vi "Process XML Node.vi"(8 "error in (no error)":errorcluster, 11 "node in":refnum<k20>) -> (0 "error out":errorcluster, 2 "Attribute":refnum<class "Attribute.lvclass">, 3 "node out":refnum<k20>)   [LabVIEW 2023, in "VILab.lvlib"]
uses:
  VILab.lvlib
  Classes/Attribute/Attribute.lvclass
  Classes/Data Item/Data Item.lvclass/Data Item.ctl
  Classes/Element/Element.lvclass/Element.ctl
  Classes/Attribute/Attribute.lvclass/Attribute.ctl
  Classes/Element Array/Element Array.lvclass
  Classes/Element/Element.lvclass
  Classes/Reference/Reference.lvclass
  Classes/Reference/Create Reference.vi
  Classes/Data Item/Data Item.lvclass
  Classes/Attribute/Create Attribute (Data Item).vi
  <vilib>/xml/NI_XML.lvlib
  <resource>/objmgr/DOMUserDefRef.rc
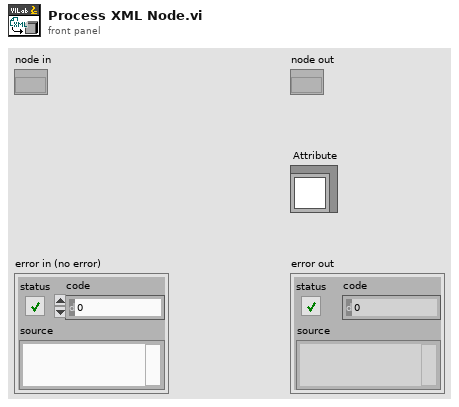
[diagram p1: front panel]
types:
  T1 = cluster{"class":string, "uid":string, "Attributes":refnum<class "Attribute.lvclass">[], "Array?":bool}
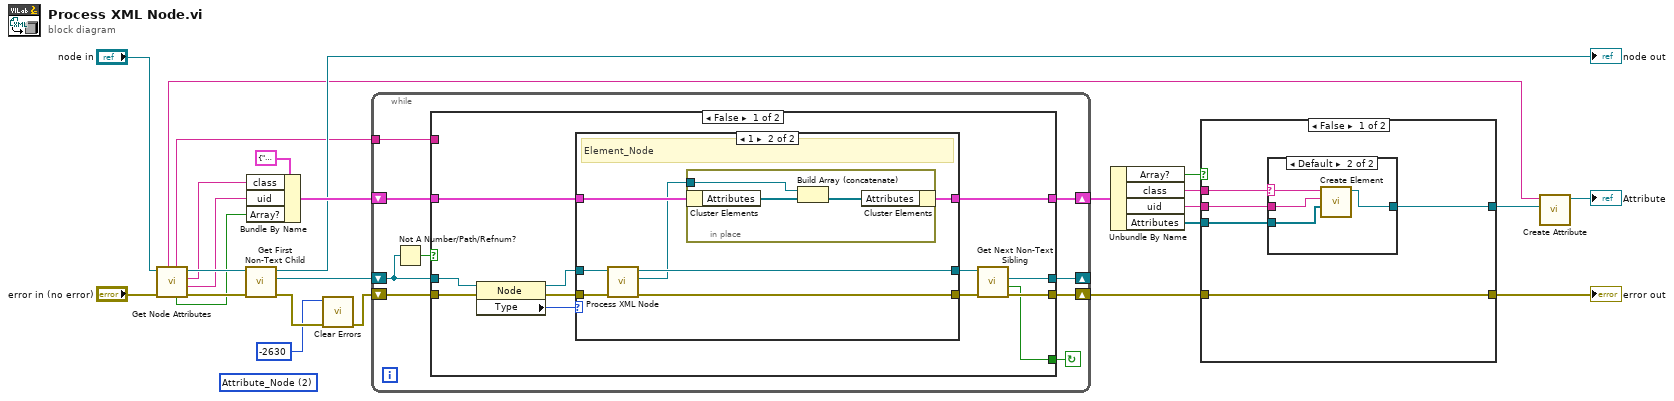
[diagram p0: block diagram]
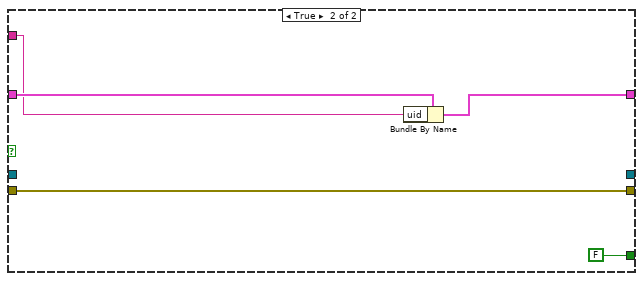
[diagram p3: hidden frame]
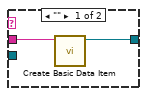
[diagram p4: hidden frame]
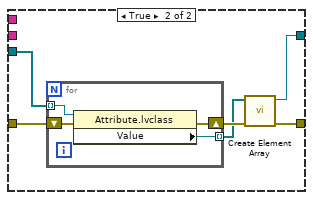
[diagram p5: hidden frame]
diagram:
  (unwired) 2 items=["Element_Node"=1, "Attribute_Node"=2, "Text_Node"=3, "CDATASection_Node"=4, "EntityReference_Node"=5, "Entity_Node"=6, "ProcessingInstruction_Node"=7, "Comment_Node"=8, "Document_Node"=9, "DocumentType_Node"=10, "DocumentFragment_Node"=11, "Notation_Node"=12] ("Node Type")
  n1 = call "Get Node Attributes.vi"("error in (no error)"="error in (no error)", "node in"="node in") -> ("error out"=w25:errorcluster, "uid"=w12:string, "class"=w13:string, "node out"=w15:refnum<k20>, "Array?"=w8:bool, "Value"=w1:string, "Name"=w2:string)  [unwired: 3 in]
  n2 = call <vilib>:"Get First Non-Text Child.vi"("error in (no error)"=w25, "node in"=w15) -> ("error out"=w23:errorcluster, "child node"=w19:refnum<k20>, "node out"=→"node out":refnum<k20>)  [unwired: 6 in, 1 out]
  n3 = Bundle By Name(cluster=T1 {"class"="", "uid"="", "Attributes"=[], "Array?"=FALSE}, "class"=w13, "uid"=w12, "Array?"=w8) -> (w11:T1)
  n4 = call <vilib>:"Clear Errors.vi"("error in (no error)"=w23, "specific error code to clear (0: all)"=-2630) -> ("error out"=w22:errorcluster)  [unwired: 4 in, 1 out]
  n5 = while {
    shift-right: [w30] -> w18
    shift-left: w11 -> [w31]
    shift-right: [w34] -> w21
    shift-left: w22 -> [w33]
    shift-right: [w29] -> _
    shift-left: w19 -> [w27]
    tunnel: w1 -> [w26]
    stop <- w32 continue-if-true
    n6 = Not A Number/Path/Refnum?(number/path/refnum=w27) -> (NaN/Path/Refnum?=w28:bool)
    n7 = case shown="False" w28 {
      tunnel: [w46 w64] -> w34
      tunnel: [w42 FALSE ("found sibling node?")] -> w32
      tunnel: w27 -> [w41 _]
      tunnel: w33 -> [w45 w64]
      tunnel: w31 -> [w38 w62]
      tunnel: [w37 w61] -> w30
      tunnel: [w36 _] -> w29
      tunnel: w26 -> [_ w60]
      frame False {
        n8 = property class="Node"(reference=w41, error in=w45) -> (reference out=w39:refnum<k20>, error out=w44:errorcluster, "Type"=w40:i32)
        n9 = case shown="1" w40 {
          tunnel: w44 -> [w49 w56]
          tunnel: w39 -> [w47 w52]
          tunnel: w38 -> [w48 w54]
          tunnel: [w48 w53] -> w37
          tunnel: [w49 w55] -> w43
          tunnel: [w47 w51] -> w35
          frame Default {
          }
          frame 1 {
            # "Element_Node"
            n10 = call "Process XML Node.vi"("error in (no error)"=w56, "node in"=w52) -> ("error out"=w55:errorcluster, "Attribute"=w50:refnum<class "Attribute.lvclass">, "node out"=w51:refnum<k20>)  [unwired: 7 in]
            n11 = in-place {
              in-place-border: w50 -> [w57]
              n12 = in-place-cluster #1(w54) -> ("Attributes"=w59:refnum<class "Attribute.lvclass">[])
              n13 = Build Array (concatenate)(w57, w59) -> (w58:refnum<class "Attribute.lvclass">[])
              n14 = in-place-cluster #1("Attributes"=w58) -> (w53:T1)
            }
          }
        }
        n15 = call <vilib>:"Get Next Non-Text Sibling.vi"("error in (no error)"=w43, "node in"=w35) -> ("error out"=w46:errorcluster, "found sibling node?"=w42:bool, "sibling node"=w36:refnum<k20>)  [unwired: 6 in, 1 out]
      }
      frame True {
        n16 = Bundle By Name(cluster=w62, "uid"=w60) -> (w61:T1)
      }
    }
  }
  n17 = Unbundle By Name(w18) -> ("Array?"=w4:bool, "class"=w5:string, "uid"=w6:string, "Attributes"=w10:refnum<class "Attribute.lvclass">[])
  n18 = case shown="False" w4 {
    tunnel: [w68 w78] -> w17
    tunnel: w6 -> [w67 _]
    tunnel: w5 -> [w66 _]
    tunnel: w10 -> [w65 w77]
    tunnel: w21 -> [w69 w81]
    tunnel: [w69 w79] -> w20
    frame False {
      n19 = case shown="Default" w66 {
        selector: w66 -> [_ w73]
        tunnel: w67 -> [w71 w75]
        tunnel: [w70 w74] -> w68
        tunnel: w65 -> [_ w72]
        frame "" {
          n20 = call "Create Basic Data Item.vi"("Content"=w71) -> ("New Data Item"=w70:refnum<class "Data Item.lvclass">)  [unwired: 10 in]
        }
        frame Default {
          n21 = call "Create Element.vi"("Attributes"=w72, "uid"=w75, "class"=w73) -> ("Element"=w74:refnum<class "Element.lvclass">)  [unwired: 8 in]
        }
      }
    }
    frame True {
      n22 = for {
        tunnel: [w83] -> w76 mode=indexing
        tunnel: w77 -> [w82] mode=indexing
        shift-right: [w84] -> w80
        shift-left: w81 -> [w85]
        n23 = property class="Attribute.lvclass"(reference=w82, error in=w85) -> (error out=w84:errorcluster, "Value"=w83:refnum<class "Data Item.lvclass">)  [unwired: 1 out]
      }
      n24 = call "Create Element Array.vi"("Error in"=w80, "Contents"=w76) -> ("Error out"=w79:errorcluster, "Element Array"=w78:refnum<class "Element Array.lvclass">)  [unwired: 8 in]
    }
  }
  "error out" <- w20
  n25 = call-poly "Create Attribute.vi"("Value"=w17, "Name"=w2) -> ("Attribute"=→"Attribute":refnum<class "Attribute.lvclass">)  [unwired: 9 in]
